vi "sendValveSignalDurringExp.vi"(0 "daq_do":tag="Dev1/ai0:1", 1 "ChangeToValve":u16, 2 "CurrentValve":u16, 3 "error in":errorcluster, 4 "controls array in":refnum<vi>[](array[refnum])) -> (8 "ValveSetTo":u16, 9 "control array out":refnum<vi>[](array[refnum]), 10 "error out":errorcluster)   [LabVIEW 2019]
uses:
  <vilib>/DAQmx/write.llb/DAQmx Write (Digital 1D Bool NChan 1Samp 1Line).vi
  <vilib>/DAQmx/miscellaneous.llb/DAQmx Fill In Error Info.vi
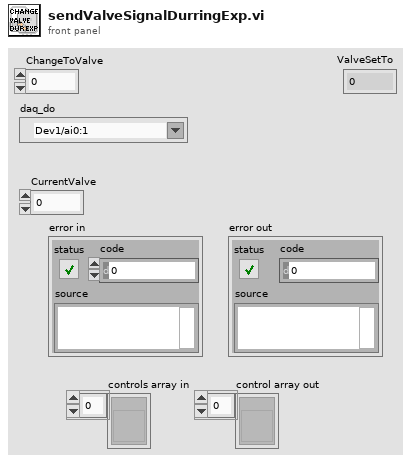
[diagram p1: front panel]
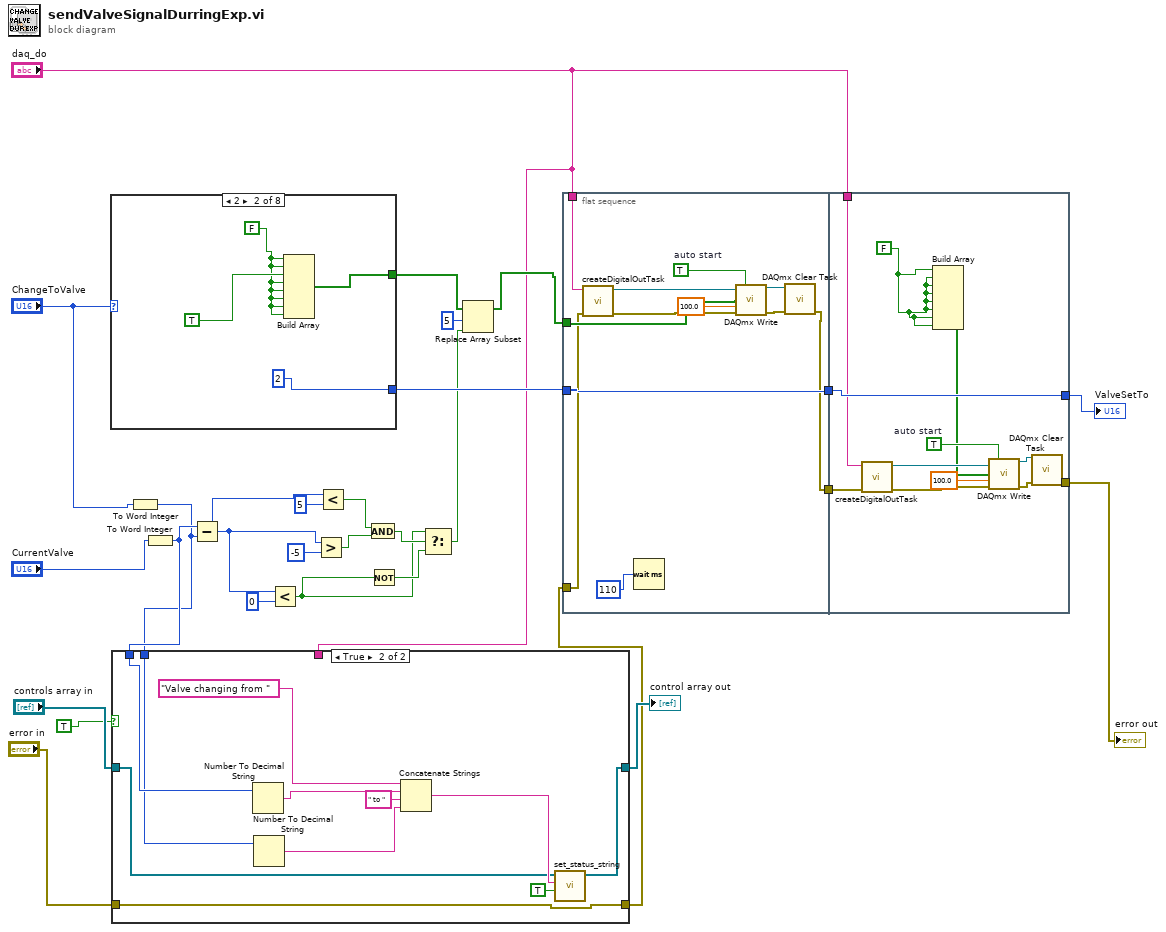
[diagram p0: block diagram]
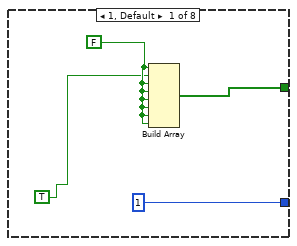
[diagram p3: hidden frame]
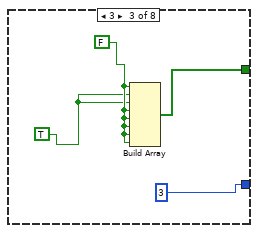
[diagram p4: hidden frame]
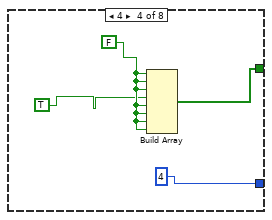
[diagram p5: hidden frame]
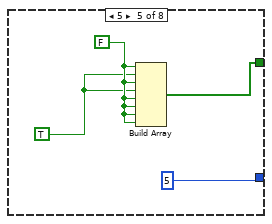
[diagram p6: hidden frame]
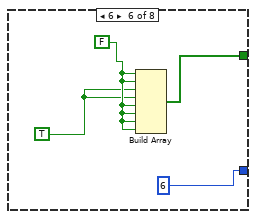
[diagram p7: hidden frame]
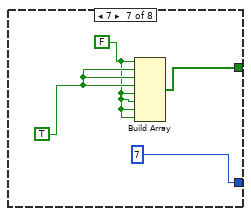
[diagram p8: hidden frame]
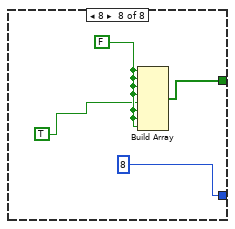
[diagram p9: hidden frame]
diagram:
  n1 = case shown="2" "ChangeToValve" {
    tunnel: [w32 w36 w40 w44 w48 w52 w56 w60] -> w14
    tunnel: [u16 1 u16 2 u16 3 u16 4 u16 5 u16 6 u16 7 u16 8] -> w28
    frame 1, Default {
      w30 = FALSE
      n2 = Build Array(w30, TRUE, w30, w30, w30, w30, w30, w30) -> (w32:bool[])
    }
    frame 2 {
      w33 = FALSE
      n3 = Build Array(w33, w33, TRUE, w33, w33, w33, w33, w33) -> (w36:bool[])
    }
    frame 3 {
      w38 = FALSE
      w37 = TRUE
      n4 = Build Array(w38, w37, w37, w38, w38, w38, w38, w38) -> (w40:bool[])
    }
    frame 4 {
      w42 = FALSE
      n5 = Build Array(w42, w42, w42, TRUE, w42, w42, w42, w42) -> (w44:bool[])
    }
    frame 5 {
      w46 = FALSE
      w45 = TRUE
      n6 = Build Array(w46, w45, w46, w45, w46, w46, w46, w46) -> (w48:bool[])
    }
    frame 6 {
      w50 = FALSE
      w49 = TRUE
      n7 = Build Array(w50, w50, w49, w49, w50, w50, w50, w50) -> (w52:bool[])
    }
    frame 7 {
      w53 = FALSE
      w54 = TRUE
      n8 = Build Array(w53, w54, w54, w54, w53, w53, w53, w53) -> (w56:bool[])
    }
    frame 8 {
      w58 = FALSE
      n9 = Build Array(w58, w58, w58, w58, TRUE, w58, w58, w58) -> (w60:bool[])
    }
  }
  n10 = To Word Integer(number="ChangeToValve") -> (16bit integer=w8:i16)
  n11 = To Word Integer(number="CurrentValve") -> (16bit integer=w9:i16)
  n12 = case shown="True" TRUE {
    tunnel: [w62 w72] -> w10
    tunnel: "controls array in" -> [w62 w64]
    tunnel: "daq_do" -> [_ _]
    tunnel: w9 -> [_ w70]
    tunnel: w8 -> [_ w67]
    tunnel: "error in" -> [w61 w63]
    tunnel: [w61 w63] -> w5
    frame False {
    }
    frame True {
      n13 = Number To Decimal String(number=w70) -> (decimal integer string=w69:string)  [unwired: 1 in]
      n14 = Number To Decimal String(number=w67) -> (decimal integer string=w66:string)  [unwired: 1 in]
      n15 = Concatenate Strings("Valve changing from ", w69, " to " ("string"), w66) -> (w65:string)
      n16 = call "set_status_string.vi"("new line?"=TRUE, "status string in"=w65, "controls array"=w64) -> ("controls array out"=w72:refnum<vi>[])  [unwired: 7 in, 1 out]
    }
  }
  "control array out" <- w10
  n17 = Subtract(x=w9, y=w8) -> (x-y=w21:i16)
  n18 = Less?(x=w21, y=i16 0) -> (x < y?=w15:bool)
  n19 = Greater?(x=w21, y=i16 -5) -> (0:w18:bool)
  n20 = Less?(x=w21, y=i16 5) -> (x < y?=w19:bool)
  n21 = And(x=w19, y=w18) -> (x .and. y?=w17:bool)
  n22 = Not(x=w15) -> (.not. x?=w16:bool)
  n23 = Select(t=w15, s=w17, f=w16) -> (s? t:f=w11:bool)
  n24 = Replace Array Subset(array=w14, new element=w11, index=5) -> (w13:bool[])
  n25 = flat-sequence {
    tunnel: "daq_do" -> [w80]
    tunnel: w13 -> [w81]
    tunnel: w28 -> [w79]
    tunnel: [w79] -> w27
    tunnel: w5 -> [w75]
    tunnel: [w74] -> w4
    tunnel: w27 -> [w97]
    tunnel: [w97] -> w26
    tunnel: "daq_do" -> [w92]
    tunnel: w4 -> [w87]
    tunnel: [w86] -> w3
    frame #0 {
      w84 = TRUE  # auto start
      n26 = call "createDigitalOutTask.vi"("error in"=w75, "daq_do"=w80) -> ("error out"=w82:errorcluster, "task out"=w83:refnum<k21>)  [unwired: 8 in]
      n27 = Wait (ms)(milliseconds to wait=u32 110) -> ()  [unwired: 1 out]
      n28 = call-poly <vilib>:"DAQmx Write.vi"("task/channels in"=w83, "auto start"=w84, "data"=w81, "timeout"=100.0, "error in"=w82) -> ("task out"=w77:refnum<k21>, "error out"=w76:errorcluster)  [unwired: 8 in, 1 out]
      n29 = call <vilib>:"DAQmx Clear Task.vi"("task in"=w77, "error in"=w76) -> ("error out"=w74:errorcluster)  [unwired: 13 in]
    }
    frame #1 {
      w90 = FALSE
      w96 = TRUE  # auto start
      n30 = call "createDigitalOutTask.vi"("error in"=w87, "daq_do"=w92) -> ("error out"=w94:errorcluster, "task out"=w95:refnum<k21>)  [unwired: 8 in]
      n31 = Build Array(w90, w90, w90, w90, w90, w90, w90, w90) -> (w93:bool[])
      n32 = call-poly <vilib>:"DAQmx Write.vi"("task/channels in"=w95, "auto start"=w96, "data"=w93, "timeout"=100.0, "error in"=w94) -> ("task out"=w89:refnum<k21>, "error out"=w88:errorcluster)  [unwired: 8 in, 1 out]
      n33 = call <vilib>:"DAQmx Clear Task.vi"("task in"=w89, "error in"=w88) -> ("error out"=w86:errorcluster)  [unwired: 13 in]
    }
  }
  "ValveSetTo" <- w26
  "error out" <- w3
